vi "Synchronize Module Events.vi"(8 "error in":errorcluster, 9 "Wait for Event Sync?":bool, 11 "Module ID in":i32) -> (0 "error out":errorcluster, 3 "Module ID out":i32)   [LabVIEW 2025, in "Data Log.lvlib"]
doc: "Call this VI to ensure the module and its caller have appropriately created and registered for events. This VI should be called after a module's caller registers for events, but before the module's caller's event structure starts. Note that registering for events is optional, but calling this VI must always be done after calling the <b>Start Module.vi</b> for a module.\n\nTo see an example of the proper wiring pattern, see the \"Run New Module: Value Change\" event frame in the API Tester VI for this module.\n_____\nBased on DQMH Dev Tools: Project Template 7.1.2.1547."
uses:
  Data Log.lvlib
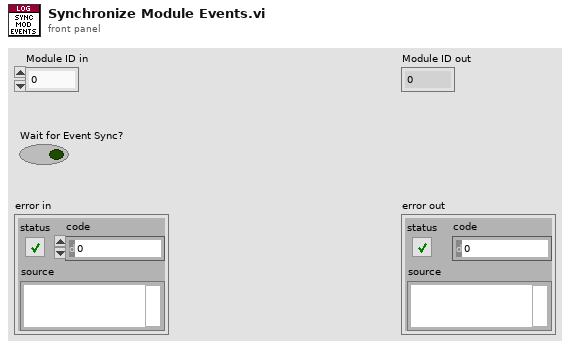
[diagram p1: front panel]
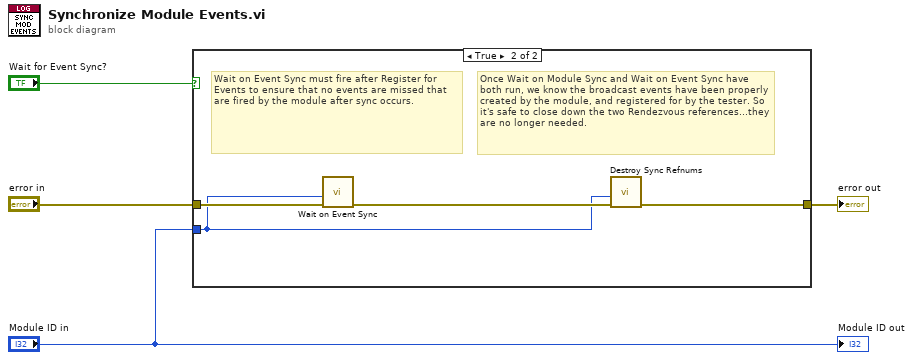
[diagram p0: block diagram]
diagram:
  n1 = case shown="True" "Wait for Event Sync?" {
    tunnel: "error in" -> [w5 w9]
    tunnel: [w5 w7] -> w3
    tunnel: "Module ID in" -> [_ w6]
    frame False {
      # "Module was already running, so the sync has already occurred elsewhere."
    }
    frame True {
      # "Once Wait on Module Sync and Wait on Event Sync have both run, we know the broadcast events have been properly created by the module, and registered for by the tester. So it's safe to close down the two Rendezvous references...they are no longer needed."
      # "Wait on Event Sync must fire after Register for Events to ensure that no events are missed that are fired by the module after sync occurs."
      n2 = call "Wait on Event Sync.vi"("error in"=w9, "Module ID"=w6) -> ("error out"=w8:errorcluster)  [unwired: 9 in]
      n3 = call "Destroy Sync Refnums.vi"("error in"=w8, "Module ID"=w6) -> ("error out"=w7:errorcluster)  [unwired: 9 in]
    }
  }
  "error out" <- w3
  "Module ID out" <- "Module ID in"
